vi "Start Blinking.vi"(11 "Blinker in":refnum<class "Blinker.lvclass">) -> (3 "Blinker out":refnum<class "Blinker.lvclass">)   [LabVIEW 2015, in "Blinker.lvclass"]
uses:
  Blinker.lvclass
  Blinker.lvclass/Blinker.ctl
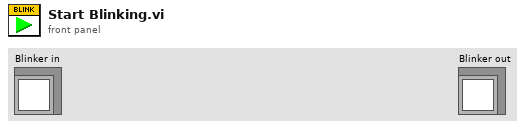
[diagram p1: front panel]
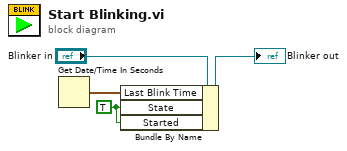
[diagram p0: block diagram]
diagram:
  w1 = TRUE ("State")
  n1 = Get Date/Time In Seconds() -> (seconds since 1Jan1904=w4:timestamp)
  n2 = Bundle By Name(cluster="Blinker in", "Last Blink Time"=w4, "State"=w1, "Started"=w1) -> (→"Blinker out":refnum<class "Blinker.lvclass">)
